vi "ping server.vi"(8 "error in":errorcluster) -> (0 "error out":errorcluster, 2 "timeout?":bool, 4 "Jl Server state out":T3, 5 "return code":u8, 6 "detailed error info":T1)   [LabVIEW 2018, in "LV-0mq-Julia_roundtrip-lib.lvlib"]
uses:
  Server or client state.ctl
  detailed error info.ctl
  StackFrame.ctl
  commands LV2Jl.ctl
  expected server response.ctl
  Commands.ctl
  ZMQ timeouts global.vi
  LV-0mq-Julia_roundtrip-lib.lvlib
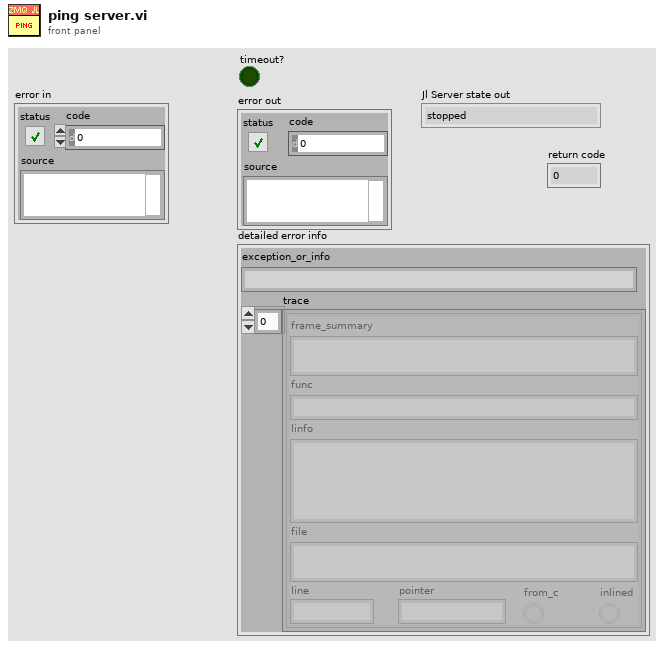
[diagram p1: front panel]
types:
  T1 = typedef "LV-0mq-Julia_roundtrip-lib.lvlib/detailed error info.ctl" = cluster{"exception_or_info":string, "trace":T2[]}
  T2 = typedef "LV-0mq-Julia_roundtrip-lib.lvlib/StackFrame.ctl" = cluster{"frame_summary":string, "func":string, "linfo":string, "file":string, "line":i32, "pointer":u64, "from_c":bool, "inlined":bool}
  T3 = typedef "LV-0mq-Julia_roundtrip-lib.lvlib/Server or client state.ctl" = enum16{"stopped", "running", "unknown"}
  T4 = typedef "LV-0mq-Julia_roundtrip-lib.lvlib/Commands.ctl" = enum16{"Start Jl-server & Init LV-client", "Send request & Get response ", "Stop Jl-server & Cleanup LV-client", "Cleanup LV-client", "Start Jl-server", "Stop Jl-server", "Init LV-Client", "Cleanup LV-Client", "(not allowed)", "Set LV Client state", "Set Jl Server state", "set ZMQ timeout", "read ZMQ timeout", "read-out state"}
  T5 = typedef "expected server response.ctl" = u16
  T6 = typedef "LV-0mq-Julia_roundtrip-lib.lvlib/commands LV2Jl.ctl" = u8
  T7 = typedef "LV-0mq-Julia_roundtrip-lib.lvlib/ZMQ timeouts.ctl" = cluster{"SNDTIMEO":i32, "RCVTIMEO":i32}
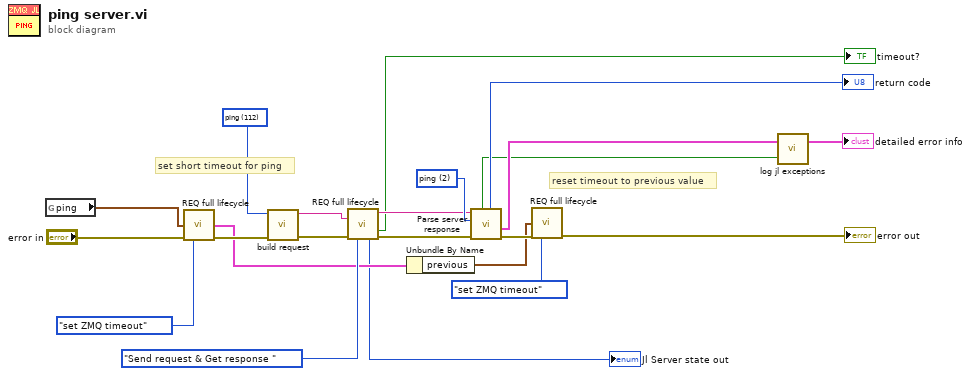
[diagram p0: block diagram]
diagram:
  w18 = T5 2 items=["detailed response", "stop", "ping"] ("expected response")
  w19 = T6 112 items=["call function"=99, "ping"=112, "stop"=115] ("Command")
  # "reset timeout to previous value"
  # "set short timeout for ping"
  n1 = global read "ZMQ timeouts global.vi" "ping"() -> (w20:T7)
  n2 = call "REQ full lifecycle.vi"("ZMQ new Timeouts in"=w20, "error in"="error in", "command"=Commands."set ZMQ timeout") -> ("ZMQ timeouts out"=w11:cluster{"previous":T7, "current":T7}, "error out"=w17:errorcluster)  [unwired: 6 in, 5 out]
  n3 = call "build request.vi"("error in (no error)"=w17, "Command"=w19) -> ("error out"=w16:errorcluster, "REQ string"=w7:string)  [unwired: 8 in]
  n4 = call "REQ full lifecycle.vi"("data to send"=w7, "error in"=w16, "command"=Commands."Send request & Get response ") -> ("server response"=w10:string, "timeout?"=→"timeout?":bool, "Jl Server state out"=→"Jl Server state out":T3, "error out"=w14:errorcluster)  [unwired: 6 in, 3 out]
  n5 = Unbundle By Name(w11) -> ("previous"=w6:T7)
  n6 = call "Parse server response.vi"("error in (no error)"=w14, "expected response"=w18, "server response in"=w10) -> ("error out"=w12:errorcluster, "detailed error info"=w3:T1, "return code"=→"return code":u8, "jl stack trace"=w1:bool)  [unwired: 1 in, 4 out]
  n7 = call "REQ full lifecycle.vi"("ZMQ new Timeouts in"=w6, "error in"=w12, "command"=Commands."set ZMQ timeout") -> ("error out"=→"error out":errorcluster)  [unwired: 6 in, 6 out]
  n8 = call "log jl exceptions.vi"("log exception"=w1, "jl error info"=w3) -> ("dup jl error info"=→"detailed error info":T1)  [unwired: 1 in]
